vi "mockbus.vi"() -> ()   [LabVIEW 2015]
uses:
  <vilib>/rvi/interface/nirviOpenFPGA/nirviOpenFPGA.xnode
  <vilib>/rvi/interface/nirviMethod/nirviMethod.xnode
  <vilib>/FPGAPlugInAG/Dynamic/niLvFpga_Abort_Dynamic.vi
  <vilib>/FPGAPlugInAG/Dynamic/niLvFpga_Run_Dynamic.vi
  <vilib>/rvi/interface/nirviCloseFPGA/nirviCloseFPGA.xnode
  <vilib>/FPGAPlugInAG/Dynamic/niLvFpga_Reset_Dynamic.vi
  Common_RT_Mockbus/Mockbus/Mockbus.lvclass
  Common_RT_Modbus/Modbus/Modbus.lvclass
  Common_RT_HealthAndStatus/RTHealthAndStatus/RTHealthAndStatus.lvclass
  Common_RT_Modbus/DataTypes/Frame.ctl
  Common_RT_Modbus/RTModbus.lvlib
  <vilib>/FPGAPlugInAG/Dynamic/niLvFpga_Close_Dynamic.vi
  MyHealthAndStatusReadFIFO/MyHealthAndStatusReadFIFO.lvclass
  MyHealthAndStatusWriteFIFO/MyHealthAndStatusWriteFIFO.lvclass
  ModbusPort1ReadFIFO/ModbusPort1ReadFIFO.lvclass
  ModbusPort1WriteFIFO/ModbusPort1WriteFIFO.lvclass
  ModbusPort2ReadFIFO/ModbusPort2ReadFIFO.lvclass
  ModbusPort2WriteFIFO/ModbusPort2WriteFIFO.lvclass
  SoftwareControlledTrigger/SoftwareControlledTrigger.lvclass
  FPGA Bitfiles/Modbus-4Port.lvbitx
  FPGA/main.vi
  <vilib>/FPGAPlugInAG/cRIO-9038/niLvFpga_Open_cRIO-9038.vi
  <vilib>/rvi/interface/common/dynamic/niFpgaDynamicAddResources.vi
panel:
  in  "Send":bool
  out "error out":errorcluster
  in  "WaitForRx":u16
  in  "Trigger?":bool
  in  "Trigger":bool
  out "Rx Data":u8[](array[numeric]) format="%02x"
  in  "Tx Data":u8[](array[numeric])=[2, 3, 64, 209] format="%02x"
  out "Port 2 Frames Received":i64
  out "Port 2 Bytes Received":i64
  out "Port 2 Frames Transmitted":i64
  out "Port 2 Bytes Transmitted":i64
  out "Port 1 Frames Received":i64
  out "Port 1 Bytes Received":i64
  out "Port 1 Frames Transmitted":i64
  out "Port 1 Bytes Transmitted":i64
  in  "Boolean":bool
  # "Port 1"
  # "Port 1 = Modbus"
  # "Port 2 = Mockbus"
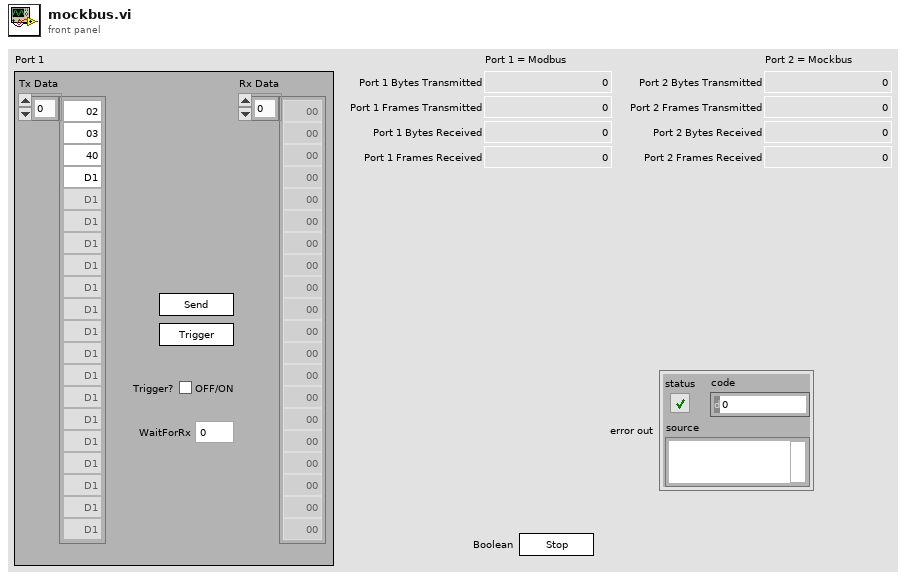
[diagram p1: front panel]
types:
  T1 = typedef "RTModbus.lvlib/Frame.ctl" = cluster{"Data":u8[], "WaitForTrigger":bool, "WaitForRx":u16, "TriggerIRQ":bool}
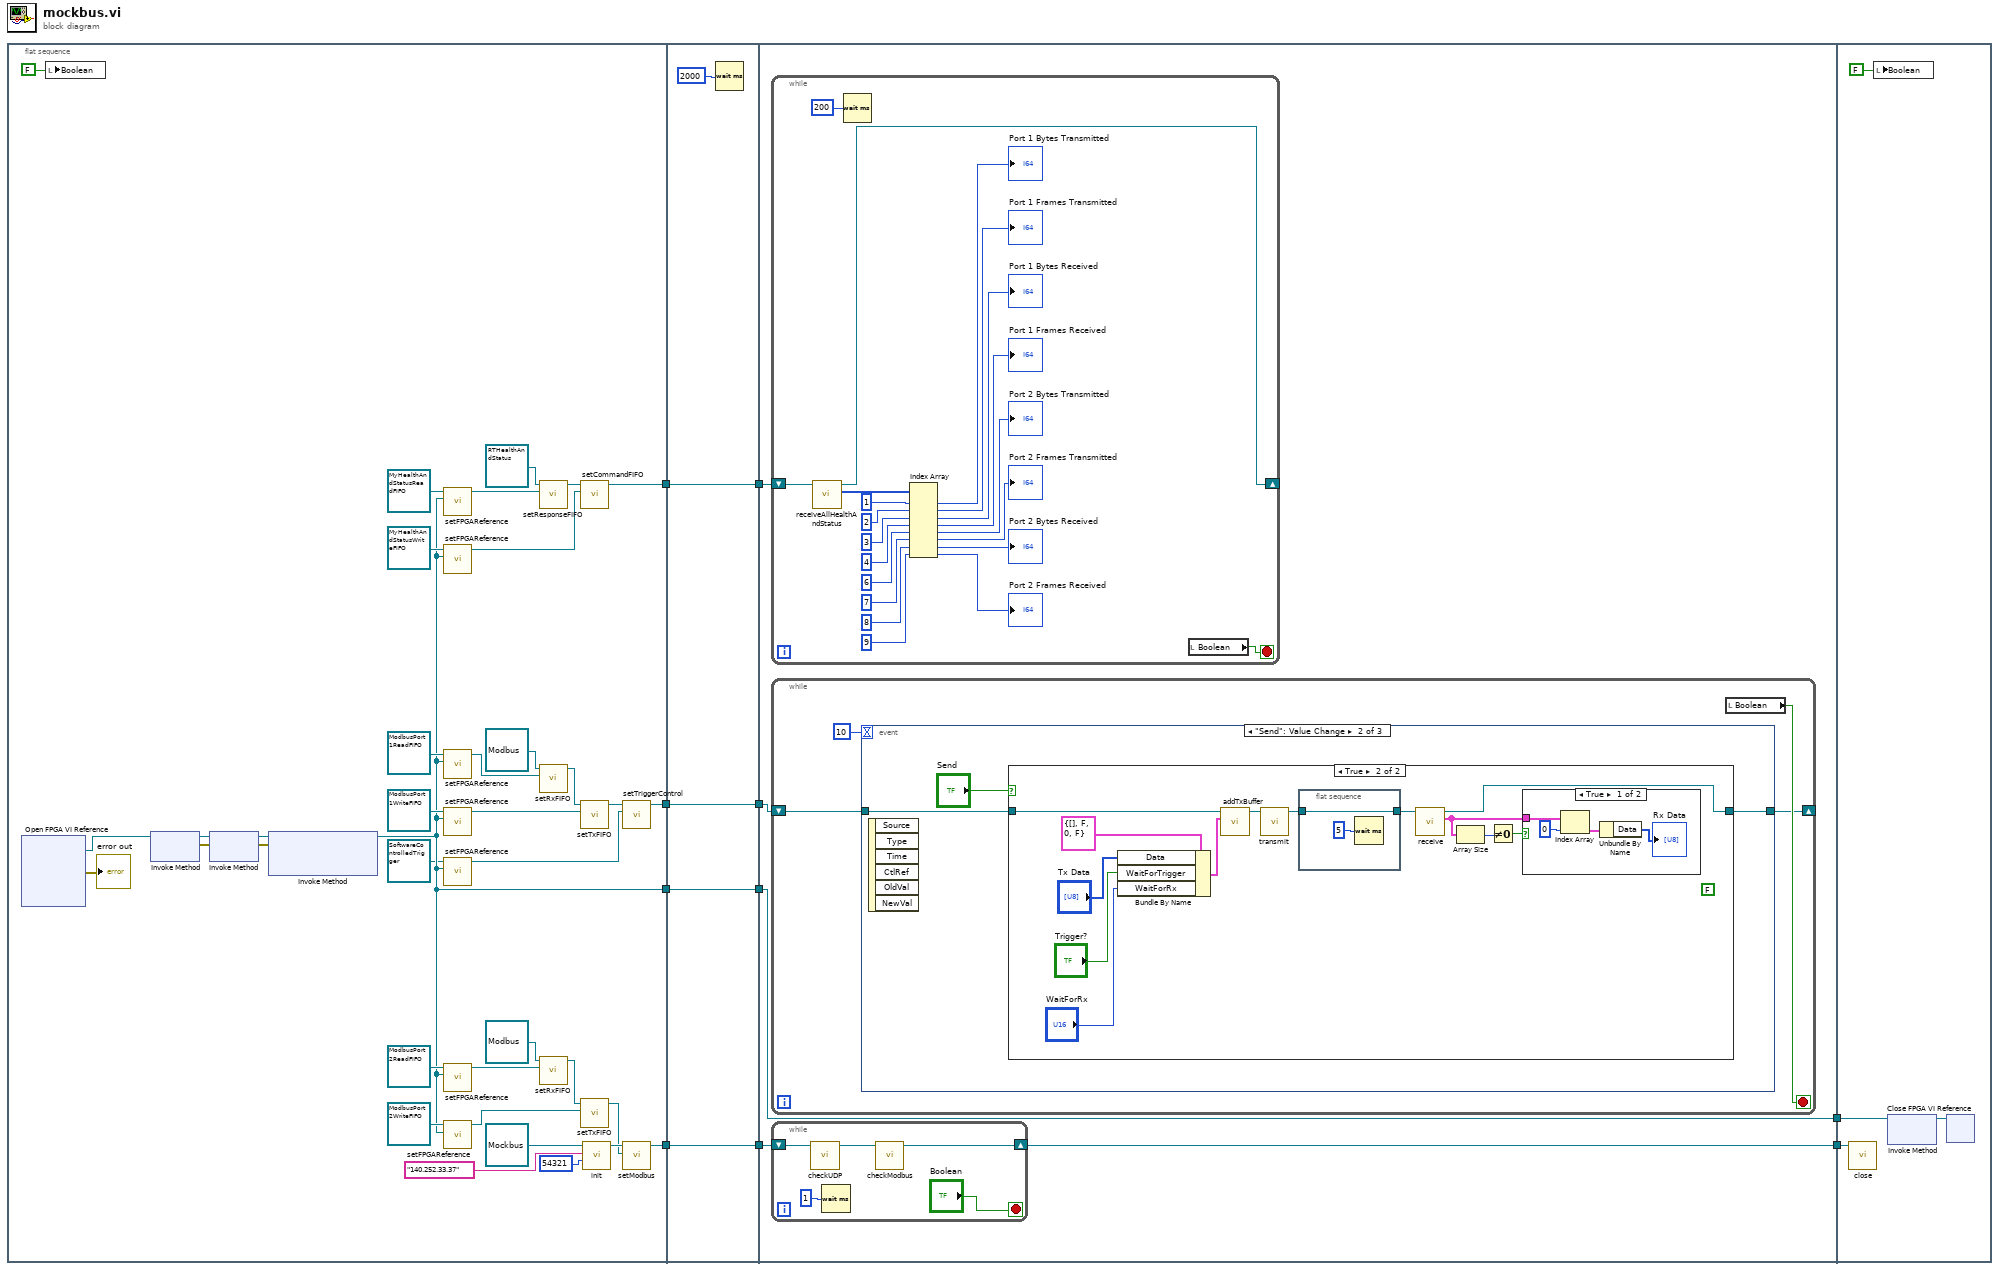
[diagram p0: block diagram]
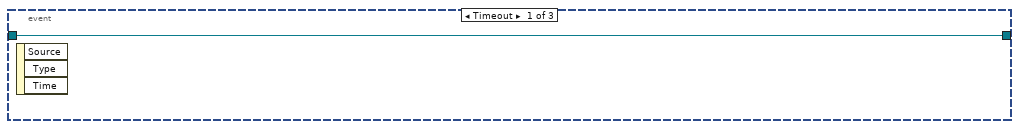
[diagram p2: hidden frame]
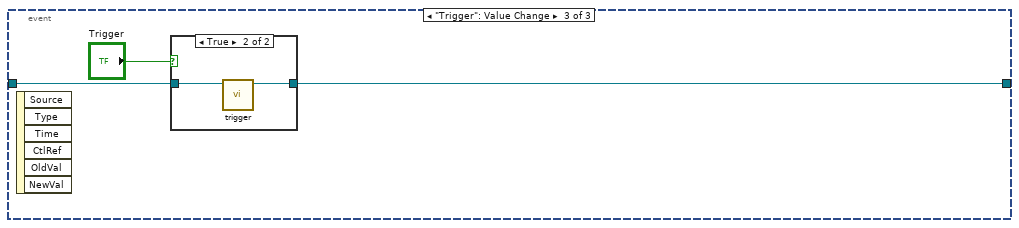
[diagram p5: hidden frame]
diagram:
  n1 = flat-sequence {
    tunnel: [w15] -> w10
    tunnel: [w41] -> w6
    tunnel: [w12] -> w4
    tunnel: [w38] -> w2
    tunnel: w10 -> [w52]
    tunnel: [w52] -> w9
    tunnel: [w50] -> w7
    tunnel: w6 -> [w50]
    tunnel: w4 -> [w49]
    tunnel: [w49] -> w3
    tunnel: w2 -> [w48]
    tunnel: [w48] -> w1
    tunnel: w9 -> [w53]
    tunnel: [w53] -> w8
    tunnel: w7 -> [w57]
    tunnel: [w56] -> w5
    tunnel: w3 -> [w55]
    tunnel: w1 -> [w54]
    tunnel: w8 -> [w120]
    tunnel: w5 -> [w119]
    frame #0 {
      n2 = xnode "Open FPGA VI Reference"() -> ("FPGA VI Reference Out"=w18:refnum<k20>, "error out"=→"error out":errorcluster)  [unwired: 2 in]
      n3 = local write "Boolean"(FALSE ("Boolean")) -> ()
      n4 = xnode "Invoke Method"("FPGA VI Reference In"=w18) -> ("FPGA VI Reference Out"=w47:refnum<k20>, "error out"=w20:errorcluster)  [unwired: 1 in]
      n5 = xnode "Invoke Method"("FPGA VI Reference In"=w47, "error in"=w20) -> ("FPGA VI Reference Out"=w46:refnum<k20>, "error out"=w19:errorcluster)
      n6 = xnode "Invoke Method"("FPGA VI Reference In"=w46, "error in"=w19) -> ("FPGA VI Reference Out"=w15:refnum<k20>)  [unwired: 1 in, 1 out]
      n7 = call "setFPGAReference.vi"("FPGAReference"=w15, "MyHealthAndStatusReadFIFO in"=refnum<class "MyHealthAndStatusReadFIFO.lvclass"> refnum ("MyHealthAndStatusReadFIFO.lvclass")) -> ("MyHealthAndStatusReadFIFO out"=w34:refnum<class "MyHealthAndStatusReadFIFO.lvclass">)  [unwired: 9 in]
      n8 = call "setFPGAReference.vi"("FPGAReference"=w15, "MyHealthAndStatusWriteFIFO in"=refnum<class "MyHealthAndStatusWriteFIFO.lvclass"> refnum ("MyHealthAndStatusWriteFIFO.lvclass")) -> ("MyHealthAndStatusWriteFIFO out"=w32:refnum<class "MyHealthAndStatusWriteFIFO.lvclass">)  [unwired: 9 in]
      n9 = call "setFPGAReference.vi"("FPGAReference"=w15, "ModbusPort1ReadFIFO in"=refnum<class "ModbusPort1ReadFIFO.lvclass"> refnum ("ModbusPort1ReadFIFO.lvclass")) -> ("ModbusPort1ReadFIFO out"=w30:refnum<class "ModbusPort1ReadFIFO.lvclass">)  [unwired: 9 in]
      n10 = call "setFPGAReference.vi"("FPGAReference"=w15, "ModbusPort1WriteFIFO in"=refnum<class "ModbusPort1WriteFIFO.lvclass"> refnum ("ModbusPort1WriteFIFO.lvclass")) -> ("ModbusPort1WriteFIFO out"=w28:refnum<class "ModbusPort1WriteFIFO.lvclass">)  [unwired: 9 in]
      n11 = call "setFPGAReference.vi"("FPGAReference"=w15, "SoftwareControlledTrigger in"=refnum<class "SoftwareControlledTrigger.lvclass"> refnum ("SoftwareControlledTrigger.lvclass")) -> ("SoftwareControlledTrigger out"=w11:refnum<class "SoftwareControlledTrigger.lvclass">)  [unwired: 9 in]
      n12 = call "setFPGAReference.vi"("FPGAReference"=w15, "ModbusPort2ReadFIFO in"=refnum<class "ModbusPort2ReadFIFO.lvclass"> refnum ("ModbusPort2ReadFIFO.lvclass")) -> ("ModbusPort2ReadFIFO out"=w22:refnum<class "ModbusPort2ReadFIFO.lvclass">)  [unwired: 9 in]
      n13 = call "setFPGAReference.vi"("FPGAReference"=w15, "ModbusPort2WriteFIFO in"=refnum<class "ModbusPort2WriteFIFO.lvclass"> refnum ("ModbusPort2WriteFIFO.lvclass")) -> ("ModbusPort2WriteFIFO out"=w23:refnum<class "ModbusPort2WriteFIFO.lvclass">)  [unwired: 9 in]
      n14 = call "setResponseFIFO.vi"("ReadU32FIFO"=w34, "RTHealthAndStatus in"=refnum<class "RTHealthAndStatus.lvclass"> refnum ("RTHealthAndStatus.lvlib:RTHealthAndStatus.lvclass")) -> ("RTHealthAndStatus out"=w39:refnum<class "RTHealthAndStatus.lvclass">)  [unwired: 9 in]
      n15 = call "setRxFIFO.vi"("ReadU16FIFO"=w30, "Modbus in"=refnum<class "Modbus.lvclass"> refnum ("RTModbus.lvlib:Modbus.lvclass")) -> ("Modbus out"=w36:refnum<class "Modbus.lvclass">)  [unwired: 9 in]
      n16 = call "setRxFIFO.vi"("ReadU16FIFO"=w22, "Modbus in"=refnum<class "Modbus.lvclass"> refnum ("RTModbus.lvlib:Modbus.lvclass")) -> ("Modbus out"=w24:refnum<class "Modbus.lvclass">)  [unwired: 9 in]
      n17 = call "setCommandFIFO.vi"("WriteU64FIFO"=w32, "RTHealthAndStatus in"=w39) -> ("RTHealthAndStatus out"=w38:refnum<class "RTHealthAndStatus.lvclass">)  [unwired: 9 in]
      n18 = call "setTxFIFO.vi"("WriteU16FIFO"=w28, "Modbus in"=w36) -> ("Modbus out"=w13:refnum<class "Modbus.lvclass">)  [unwired: 9 in]
      n19 = call "setTxFIFO.vi"("WriteU16FIFO"=w23, "Modbus in"=w24) -> ("Modbus out"=w21:refnum<class "Modbus.lvclass">)  [unwired: 9 in]
      n20 = call "init.vi"("Port"=u16 54321 ("port"), "IP"="140.252.33.37" ("name"), "Mockbus in"=refnum<class "Mockbus.lvclass"> refnum ("Mockbus.lvclass")) -> ("Mockbus out"=w42:refnum<class "Mockbus.lvclass">)  [unwired: 7 in, 1 out]
      n21 = call "setTriggerControl.vi"("TriggerControl"=w11, "Modbus in"=w13) -> ("Modbus out"=w12:refnum<class "Modbus.lvclass">)  [unwired: 9 in]
      n22 = call "setModbus.vi"("Modbus.lvclass"=w21, "Mockbus in"=w42) -> ("Mockbus out"=w41:refnum<class "Mockbus.lvclass">)  [unwired: 9 in]
    }
    frame #1 {
      n23 = Wait (ms)(milliseconds to wait=u32 2000) -> ()  [unwired: 1 out]
    }
    frame #2 {
      n24 = while {
        shift-right: [w75] -> _
        shift-left: w54 -> [w76]
        stop <- w78 stop-if-true
        n25 = call "receiveAllHealthAndStatus.vi"("RTHealthAndStatus in"=w76) -> ("Telemetry"=w70:u32[], "RTHealthAndStatus out"=w75:refnum<class "RTHealthAndStatus.lvclass">)  [unwired: 8 in, 1 out]
        n26 = Wait (ms)(milliseconds to wait=u32 200) -> ()  [unwired: 1 out]
        n27 = Index Array(array=w70, index #1=1 ("index"), index #2=2 ("index"), index #3=3 ("index"), index #4=4 ("index"), index #5=6 ("index"), index #6=7 ("index"), index #7=8 ("index"), index #8=9 ("index")) -> (element #1=→"Port 1 Bytes Transmitted":u32, element #2=→"Port 1 Frames Transmitted":u32, element #3=→"Port 1 Bytes Received":u32, element #4=→"Port 1 Frames Received":u32, element #5=→"Port 2 Bytes Transmitted":u32, element #6=→"Port 2 Frames Transmitted":u32, element #7=→"Port 2 Bytes Received":u32, element #8=→"Port 2 Frames Received":u32)
        n28 = local read "Boolean"() -> (w78:bool)
      }
      n29 = while {
        shift-right: [w79] -> _
        shift-left: w55 -> [w80]
        stop <- w82 stop-if-true
        n30 = event shown="[1] \"Send\": Value Change" {
          selector: _ -> [_ _ _]
          dyn-events: _ -> [_ _ _]
          timeout: 10 -> [_ _ _]
          tunnel: w80 -> [w83 w85 w108]
          tunnel: [w83 w84 w107] -> w79
          event Timeout {
            n31 = event-data() -> ()  [unwired: 1 in, 3 out]
          }
          event "Send": Value Change {
            n32 = event-data() -> ()  [unwired: 1 in, 6 out]
            n33 = case shown="True" "Send" {
              tunnel: w85 -> [w87 w100]
              tunnel: [w87 w93] -> w84
              frame False {
              }
              frame True {
                (unwired) FALSE ("Go!")
                n34 = Bundle By Name(cluster=T1 {"Data"=[], "WaitForTrigger"=FALSE, "WaitForRx"=0, "TriggerIRQ"=FALSE} ("Frame"), "Data"="Tx Data", "WaitForTrigger"="Trigger?", "WaitForRx"="WaitForRx") -> (w91:T1)
                n35 = call "addTxBuffer.vi"("Frame"=w91, "Modbus in"=w100) -> ("Modbus out"=w99:refnum<class "Modbus.lvclass">)  [unwired: 8 in, 1 out]
                n36 = call "transmit.vi"("Modbus in"=w99) -> ("Modbus out"=w95:refnum<class "Modbus.lvclass">)  [unwired: 9 in, 1 out]
                n37 = flat-sequence {
                  tunnel: [w101] -> w94
                  tunnel: w95 -> [w101]
                  frame #0 {
                    n38 = Wait (ms)(milliseconds to wait=u32 5) -> ()  [unwired: 1 out]
                  }
                }
                n39 = call "receive.vi"("Modbus in"=w94) -> ("Data"=w98:T1[], "Modbus out"=w93:refnum<class "Modbus.lvclass">)  [unwired: 8 in, 1 out]
                n40 = Array Size(array=w98) -> (size(s)=w97:i32)
                n41 = Not Equal To 0?(x=w97) -> (x != 0?=w96:bool)
                n42 = case shown="True" w96 {
                  tunnel: w98 -> [w106 _]
                  frame True {
                    n43 = Index Array(array=w106, index=0) -> (element=w104:T1)
                    n44 = Unbundle By Name(w104) -> ("Data"=→"Rx Data":u8[])
                  }
                  frame False {
                  }
                }
              }
            }
          }
          event "Trigger": Value Change {
            n45 = event-data() -> ()  [unwired: 1 in, 6 out]
            n46 = case shown="True" "Trigger" {
              tunnel: w108 -> [w110 w112]
              tunnel: [w110 w111] -> w107
              frame False {
              }
              frame True {
                n47 = call "trigger.vi"("Modbus in"=w112) -> ("Modbus out"=w111:refnum<class "Modbus.lvclass">)  [unwired: 9 in, 1 out]
              }
            }
          }
        }
        n48 = local read "Boolean"() -> (w82:bool)
      }
      n49 = while {
        shift-right: [w114] -> w56
        shift-left: w57 -> [w117]
        stop <- "Boolean" stop-if-true
        n50 = call "checkUDP.vi"("Mockbus in"=w117) -> ("Mockbus out"=w115:refnum<class "Mockbus.lvclass">)  [unwired: 9 in, 1 out]
        n51 = Wait (ms)(milliseconds to wait=u32 1) -> ()  [unwired: 1 out]
        n52 = call "checkModbus.vi"("Mockbus in"=w115) -> ("Mockbus out"=w114:refnum<class "Mockbus.lvclass">)  [unwired: 9 in, 1 out]
      }
    }
    frame #3 {
      n53 = call "close.vi"("Mockbus in"=w119) -> ()  [unwired: 9 in, 2 out]
      n54 = local write "Boolean"(FALSE ("Boolean")) -> ()
      n55 = xnode "Invoke Method"("FPGA VI Reference In"=w120) -> ("FPGA VI Reference Out"=w121:refnum<k20>)  [unwired: 1 in, 1 out]
      n56 = xnode "Close FPGA VI Reference"("FPGA VI Reference In"=w121) -> ()  [unwired: 1 in, 1 out]
    }
  }
